vi "performZeroCheck.vi"(6 "Mode":i32(ring) items=["Current", "Charge", "Voltage", "Resistance"], 8 "error in (no error)":errorcluster, 9 "Input Range":dbl format="%#_10g", 10 "Electrometer in":refnum<class "Electrometer.lvclass">, 11 "ReadyState in":refnum<class "ReadyState.lvclass">) -> (0 "error out":errorcluster, 1 "Range":string, 2 "Electrometer out":refnum<class "Electrometer.lvclass">, 3 "ReadyState out":refnum<class "ReadyState.lvclass">)   [LabVIEW 2016, in "ReadyState.lvclass"]
uses:
  ReadyState.lvclass
  Electrometer.lvclass
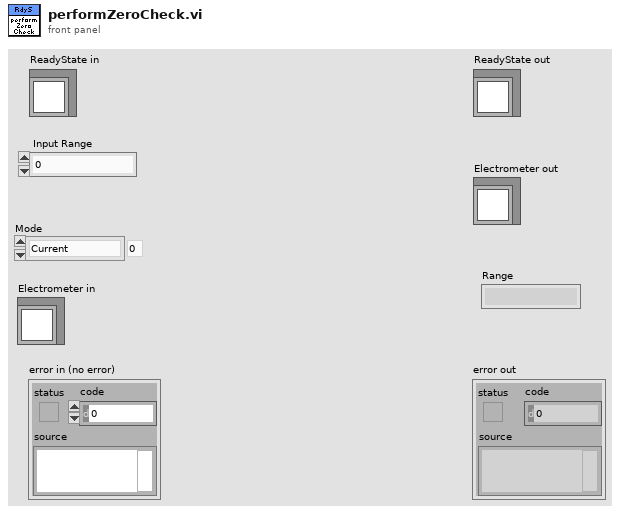
[diagram p1: front panel]
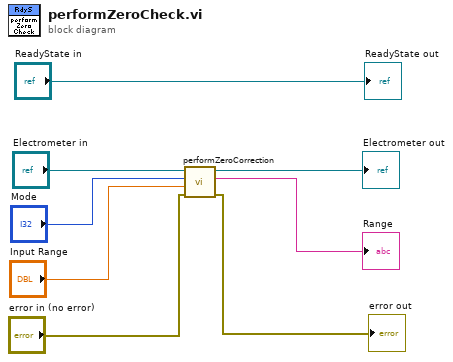
[diagram p0: block diagram]
diagram:
  n1 = call "performZeroCorrection.vi"("error in (no error)"="error in (no error)", "Input Range"="Input Range", "Measurement Function (0: Current)"="Mode", "Electrometer in"="Electrometer in") -> ("error out"=→"error out":errorcluster, "Set Range"=→"Range":string, "Electrometer out"=→"Electrometer out":refnum<class "Electrometer.lvclass">)  [unwired: 5 in]
  "ReadyState out" <- "ReadyState in"
